vi "ScanDelay_FTIR_GetSpectrum_Aligning.vi"(0 "Cancel? External":refnum<vi>, 1 "% averaged (external)":refnum<vi>, 2 "Binned interferogram (external)":refnum<vi>, 3 "Python refnum in":refnum<k35>, 5 "Optimize\ninterferogram\ndelay":bool, 7 "Acquisition cycle (external)":refnum<vi>, 8 "Fmin / Fmax":T1={"Min frequency"=800.0, "Max frequency"=2500.0}, 9 "Displacement\n calibration  factor":dbl=-2.438, 10 "Python error in":errorcluster, 11 "Channels to read  (ScanDelay X, chan(1,2,..))":tag="Dev1/ai3,Dev1/ai2,Dev1/ai2", 12 "Acquisitions per interferogram":i32=30, 13 "Time per\nacquisition (s)":dbl=0.18, 14 "Sampling rate":dbl=250000.0, 15 "Delay estimation (pts)":i32=-10) -> (4 "Output spectrum":dbl[][](array[numeric]), 6 "Best delay":i32)   [LabVIEW 2022 SP3]
uses:
  Control_GetSpectrum_Aligning.ctl
  <vilib>/DAQmx/read.llb/DAQmx Read (Analog 2D DBL NChan NSamp).vi
  <vilib>/DAQmx/miscellaneous.llb/DAQmx Fill In Error Info.vi
panel:
  out "size(s)":i32[](array[numeric])
  out "Number of signal channels":i32
  in  "Gain":dbl=1.0
  in  "First clear existing DAQmx tasks":bool=TRUE
  in  "Optimize over delay range":i32=5
  in  "Flattening order":i32=5
  out "DAQmx error":errorcluster={"status"=FALSE, "code"=200012, "source"="DAQmx Control Task.vi:3900003"}
  out "Time per\nloop (ms)":dbl=199.0
  in  "Save interferograms\n(interferograms.txt)":bool=TRUE
  out "Own python session":bool
  in  "Extract envelope":bool=TRUE
  out "Refnum errors":errorcluster
  out "Spectrum (amplitude)":cluster{dbl[], dbl[]}[](graph)
  out "Spectrum (phase)":cluster{dbl[], dbl[]}[](graph)
  out "Interferogram (aligned)":cluster{dbl[], dbl[]}[](graph)
  out "% averaged":dbl=46.666666666666664
  out "Acquisition cycle":dbl[][](graph)
  out "Python error out":errorcluster
  in  "Halt acquisition":bool
  in  "Subtract\ndisplacement (ps)":dbl
  out "Python module path":path=path "C:/Users/mnopl/Desktop/Software/mnOPSuite/PRISM/python/scandelay_FTIR.py"
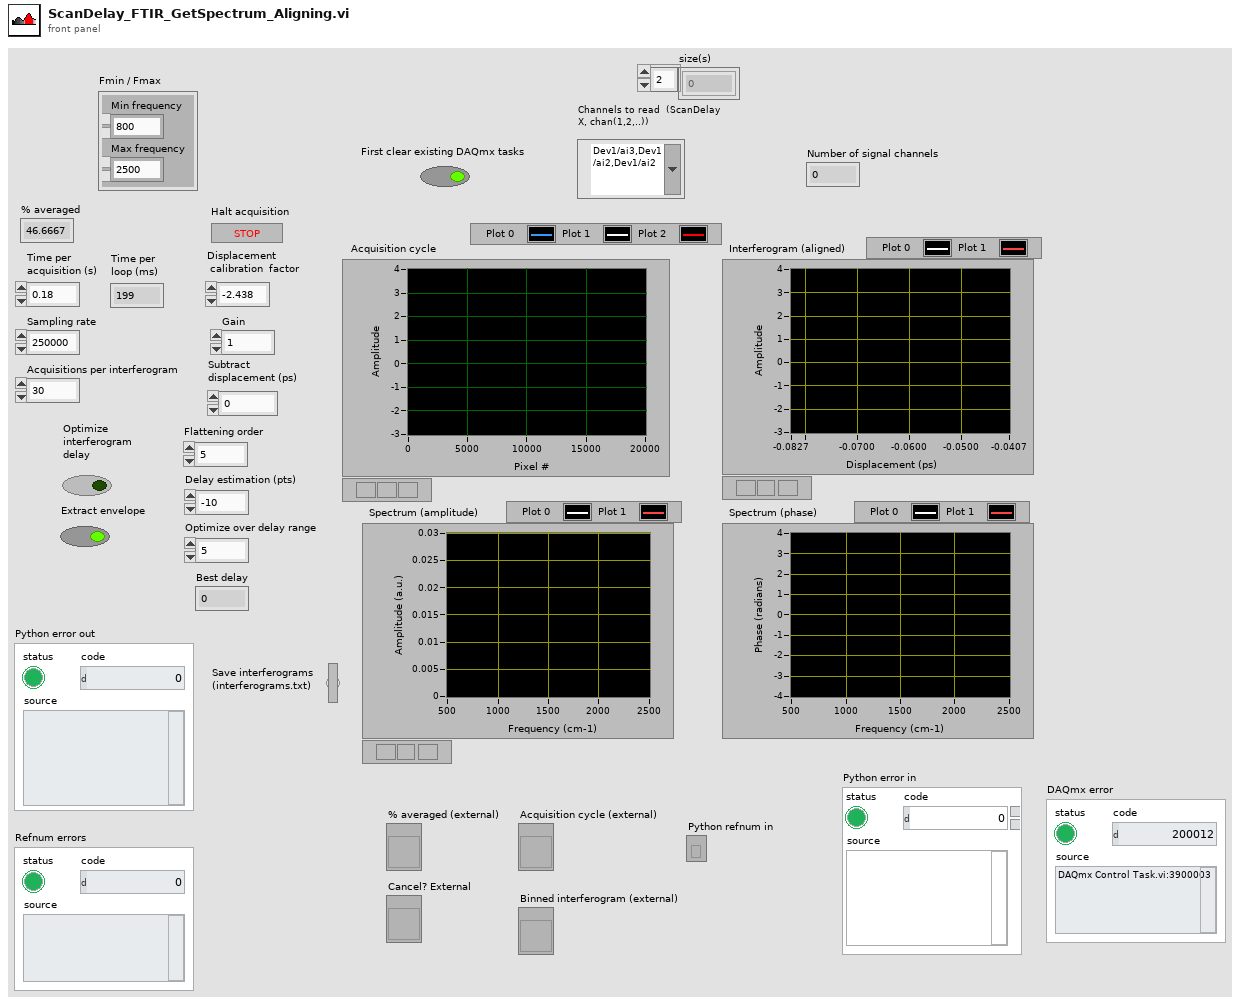
[diagram p1: front panel]
types:
  T1 = cluster{"Min frequency":dbl, "Max frequency":dbl}
  T2 = typedef "Control_GetSpectrum_Aligning.ctl" = enum16{"Acquire Interferograms", "Prepare DAQ task", "Align Interferograms", "Compute Spectrum", "Done"}
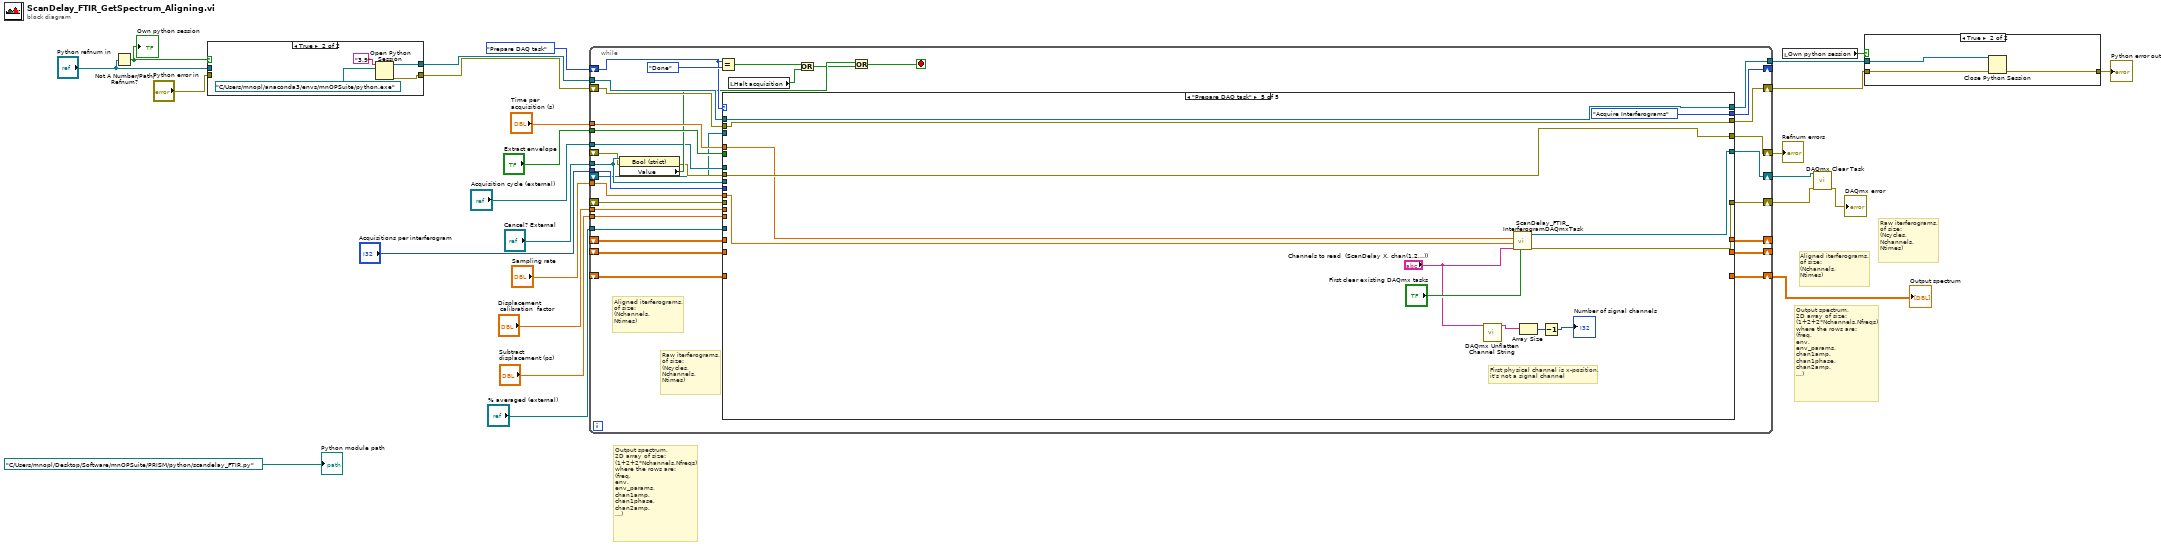
[diagram p0: block diagram]
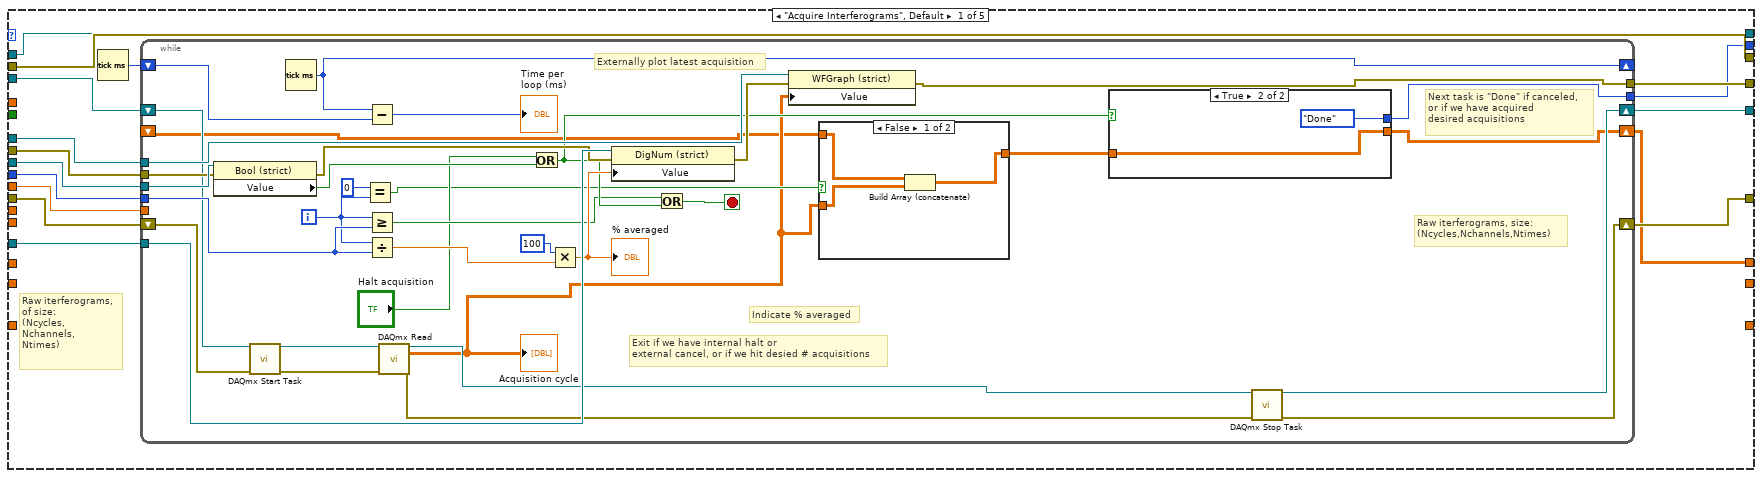
[diagram p4: hidden frame]
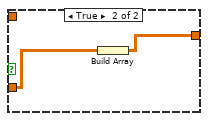
[diagram p5: hidden frame]
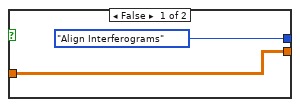
[diagram p6: hidden frame]
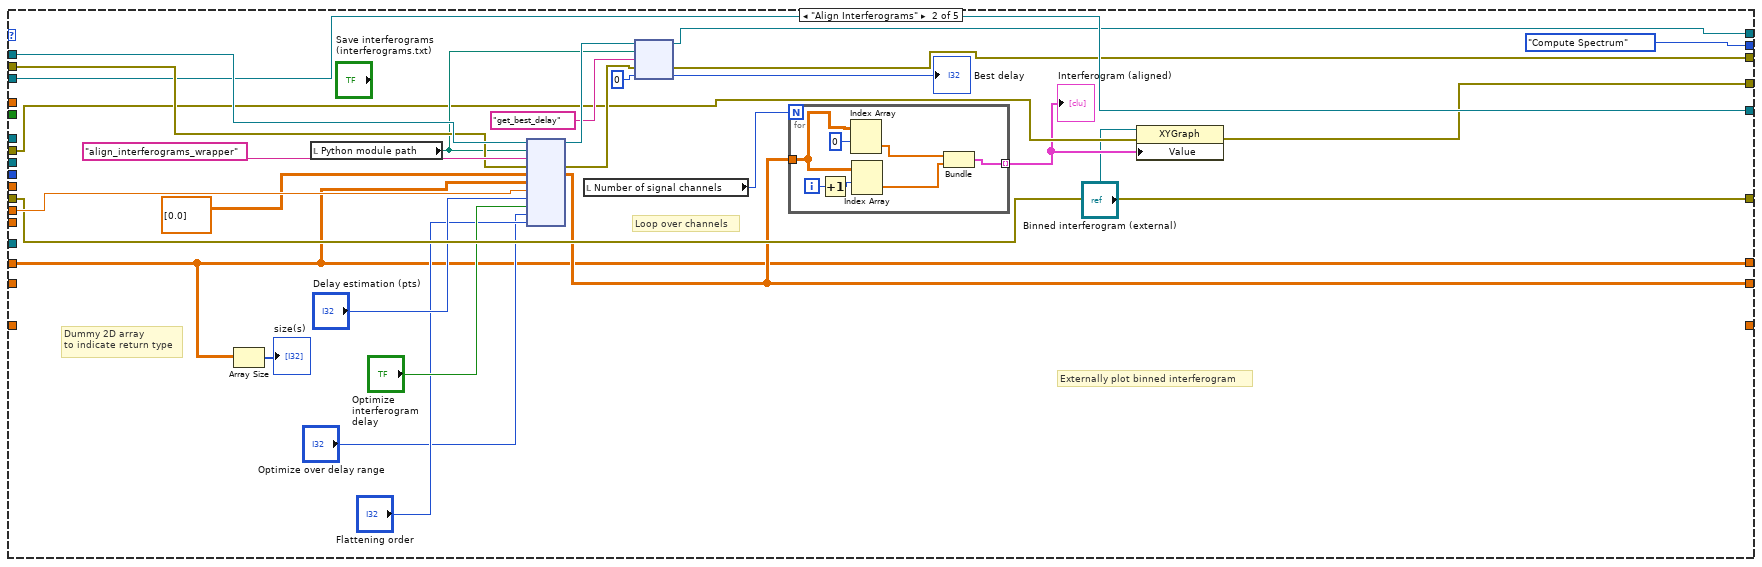
[diagram p7: hidden frame]
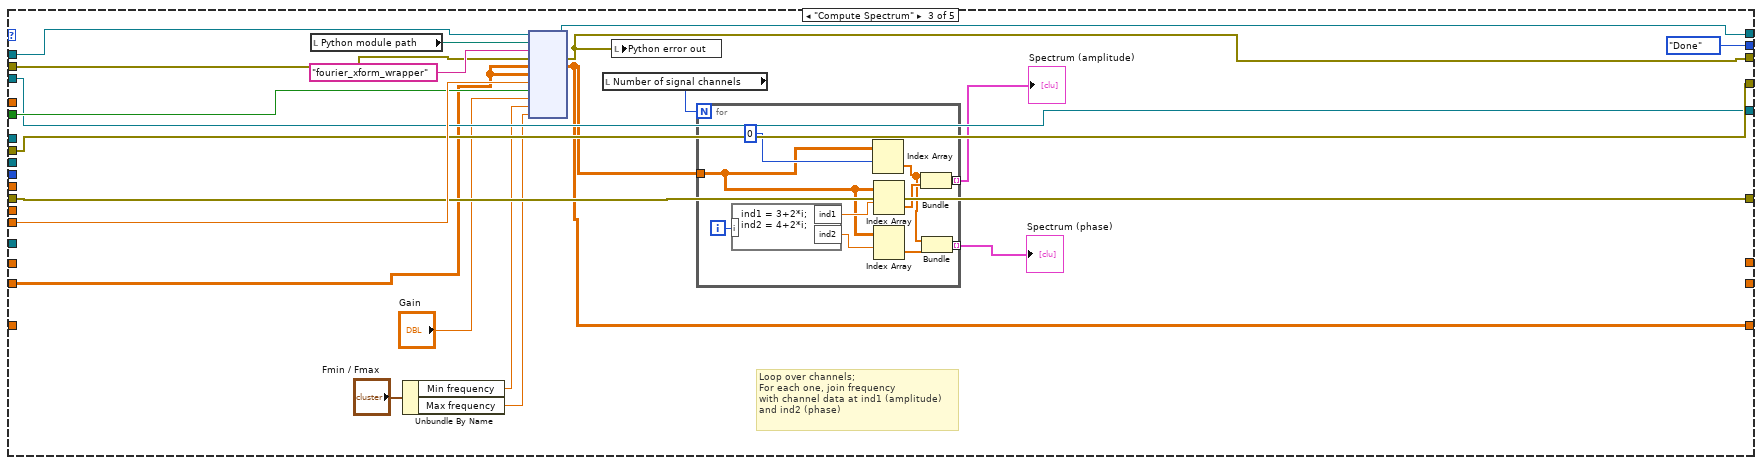
[diagram p8: hidden frame]
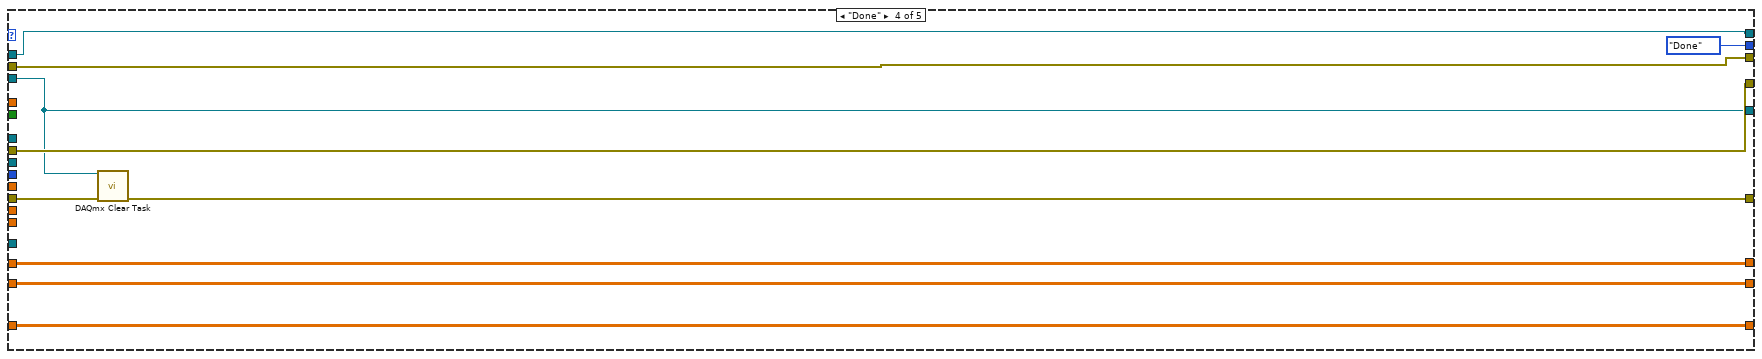
[diagram p9: hidden frame]
diagram:
  # "Output spectrum,\n2D array of size:\n(1+2+2*Nchannels,Nfreqs)\nwhere the rows are:\n(freq,\nenv,\nenv_params,\nchan1amp,\nchan1phase,\nchan2amp,\n...)"
  # "Output spectrum,\n2D array of size:\n(1+2+2*Nchannels,Nfreqs)\nwhere the rows are:\n(freq,\nenv,\nenv_params,\nchan1amp,\nchan1phase,\nchan2amp,\n...)"
  # "Aligned iterferograms,\nof size:\n(Nchannels,\nNtimes)"
  # "Raw iterferograms,\nof size:\n(Ncycles,\nNchannels,\nNtimes)"
  n1 = Not A Number/Path/Refnum?(number/path/refnum="Python refnum in") -> (NaN/Path/Refnum?=w7:bool)
  "Own python session" <- w7
  n2 = case shown="True" w7 {
    tunnel: [w27 w29] -> w11
    tunnel: [w26 w28] -> w10
    tunnel: "Python refnum in" -> [w27 _]
    tunnel: "Python error in" -> [w26 _]
    frame False {
    }
    frame True {
      n3 = Open Python Session(python version="3.9", python path=path "C:/Users/mnopl/anaconda3/envs/mnOPSuite/python.exe") -> (session out=w29:refnum<k35>, error out=w28:errorcluster)  [unwired: 1 in]
    }
  }
  n4 = while {
    tunnel: w11 -> [w65]
    tunnel: "Acquisition cycle (external)" -> [w42]
    tunnel: "Sampling rate" -> [w63]
    tunnel: "Time per\nacquisition (s)" -> [w62]
    tunnel: "Displacement\n calibration  factor" -> [w61]
    tunnel: "% averaged (external)" -> [w60]
    tunnel: "Cancel? External" -> [w45]
    tunnel: "Acquisitions per interferogram" -> [w59]
    shift-right: [w58] -> _
    shift-left: Control_GetSpectrum_Aligning."Prepare DAQ task" -> [w50]
    tunnel: "Subtract\ndisplacement (ps)" -> [w57]
    tunnel: [w54] -> w15
    shift-right: [w53] -> w14
    shift-left: w10 -> [w64]
    tunnel: "Extract envelope" -> [w52]
    shift-right: [w51] -> w12
    shift-left: _ -> [w43]
    shift-right: [w40] -> w4
    shift-left: _ -> [w38]
    shift-right: [w41] -> w2
    shift-left: _ -> [w39]
    shift-right: [w37] -> _
    shift-left: _ -> [w36]
    shift-right: [w35] -> _
    shift-left: _ -> [w34]
    shift-right: [w33] -> w1
    shift-left: _ -> [w32]
    stop <- w47 stop-if-true
    # "Aligned iterferograms,\nof size:\n(Nchannels,\nNtimes)"
    # "Raw iterferograms,\nof size:\n(Ncycles,\nNchannels,\nNtimes)"
    n5 = property on="Property Node" class="Bool (strict)"(reference=w45, error in=w43) -> (error out=w44:errorcluster, "Value"=w49:bool)  [unwired: 1 out]
    n6 = Equal?(x=w50, y=Control_GetSpectrum_Aligning."Done") -> (x = y?=w55:bool)
    n7 = case shown="\"Prepare DAQ task\"" w50 {
      tunnel: w65 -> [w68 w152 w180 w200 w210]
      tunnel: w64 -> [w77 w151 w177 w201 w209]
      tunnel: w42 -> [w81 _ _ _ _]
      tunnel: w63 -> [w80 _ _ _ w207]
      tunnel: w62 -> [_ _ _ _ w208]
      tunnel: w61 -> [_ w149 _ _ _]
      tunnel: w60 -> [w79 _ _ _ _]
      tunnel: w45 -> [w78 _ _ _ _]
      tunnel: w59 -> [w75 _ _ _ _]
      tunnel: [w68 w141 w179 w200 w210] -> w54
      tunnel: [w73 Control_GetSpectrum_Aligning."Compute Spectrum" Control_GetSpectrum_Aligning."Done" Control_GetSpectrum_Aligning."Done" Control_GetSpectrum_Aligning."Acquire Interferograms"] -> w58
      tunnel: w57 -> [_ _ w176 _ _]
      tunnel: [w77 w139 w173 w201 w209] -> w53
      tunnel: w52 -> [_ _ w174 _ _]
      tunnel: [w76 w131 w172 w198 w212] -> w51
      tunnel: w44 -> [w74 w132 w172 w198 w212]
      tunnel: [w70 w148 w171 w197 w214] -> w41
      tunnel: [w69 w147 w170 w195 w213] -> w40
      tunnel: w39 -> [w72 w148 w171 w197 _]
      tunnel: w38 -> [w71 w147 w170 w196 _]
      tunnel: [w66 w127 _ w192 _] -> w37
      tunnel: w36 -> [_ w127 _ w192 _]
      tunnel: [_ w133 _ w193 _] -> w35
      tunnel: w34 -> [_ _ w165 w193 _]
      tunnel: [_ _ w164 w194 _] -> w33
      tunnel: w32 -> [_ _ _ w194 _]
      frame "Acquire Interferograms", Default {
        # "Raw iterferograms,\nof size:\n(Ncycles,\nNchannels,\nNtimes)"
        n8 = Tick Count (ms)() -> (millisecond timer value=w67:u32)
        n9 = while {
          tunnel: w81 -> [w112]
          tunnel: w80 -> [_]
          tunnel: w79 -> [w114]
          tunnel: w78 -> [w109]
          tunnel: [w110] -> w76
          shift-right: [w88] -> w66
          shift-left: _ -> [w83]
          tunnel: w75 -> [w103]
          tunnel: w74 -> [w108]
          tunnel: [w105] -> w73
          shift-right: [w100] -> w70
          shift-left: w72 -> [w91]
          shift-right: [w101] -> w69
          shift-left: w71 -> [w90]
          shift-right: [w99] -> _
          shift-left: w67 -> [w98]
          i -> [w87]
          stop <- w106 stop-if-true
          # "Raw iterferograms, size:\n(Ncycles,Nchannels,Ntimes)"
          # "Next task is \"Done\" if canceled,\nor if we have acquired \ndesired acquisitions"
          # "Exit if we have internal halt or\nexternal cancel, or if we hit desied # acquisitions"
          # "Externally plot latest acquisition"
          # "Indicate % averaged"
          n10 = property on="Property Node" class="Bool (strict)"(reference=w109, error in=w108) -> (error out=w107:errorcluster, "Value"=w104:bool)  [unwired: 1 out]
          n11 = call <vilib>:"DAQmx Start Task.vi"("task/channels in"=w91, "error in"=w90) -> ("task out"=w92:refnum<k21>, "error out"=w89:errorcluster)  [unwired: 12 in]
          n12 = Tick Count (ms)() -> (millisecond timer value=w99:u32)
          n13 = Equal?(x=0, y=w87) -> (x = y?=w85:bool)
          n14 = Subtract(x=w99, y=w98) -> (x-y=→"Time per\nloop (ms)":u32)
          n15 = Greater Or Equal?(x=w87, y=w103) -> (x >= y?=w95:bool)
          n16 = Divide(x=w87, y=w103) -> (x/y=w116:dbl)
          n17 = call-poly <vilib>:"DAQmx Read.vi"("task/channels in"=w92, "error in"=w89) -> ("task out"=w93:refnum<k21>, "data"=w84:dbl[][], "error out"=w102:errorcluster)  [unwired: 11 in]
          "Acquisition cycle" <- w84
          n18 = Or(x="Halt acquisition", y=w104) -> (x .or. y?=w96:bool)
          n19 = Multiply(x=100, y=w116) -> (x*y=w113:dbl)
          "% averaged" <- w113
          n20 = property on="Property Node" class="DigNum (strict)"(reference=w114, error in=w107, "Value"=w113) -> (error out=w111:errorcluster)  [unwired: 1 out]
          n21 = Or(x=w95, y=w96) -> (x .or. y?=w106:bool)
          n22 = property on="Property Node" class="WFGraph (strict)"(reference=w112, error in=w111, "Value"=w84) -> (error out=w110:errorcluster)  [unwired: 1 out]
          n23 = case shown="False" w85 {
            tunnel: w84 -> [w118 w121]
            tunnel: w83 -> [w119 _]
            tunnel: [w117 w120] -> w82
            frame False {
              n24 = Build Array (concatenate)(w119, w118) -> (w117:dbl[][][])
            }
            frame True {
              n25 = Build Array(w121) -> (w120:dbl[][][])
            }
          }
          n26 = case shown="True" w96 {
            tunnel: [Control_GetSpectrum_Aligning."Align Interferograms" Control_GetSpectrum_Aligning."Done"] -> w105
            tunnel: [w122 w124] -> w88
            tunnel: w82 -> [w122 w124]
            frame False {
            }
            frame True {
            }
          }
          n27 = call <vilib>:"DAQmx Stop Task.vi"("task/channels in"=w93, "error in"=w102) -> ("task out"=w100:refnum<k21>, "error out"=w101:errorcluster)  [unwired: 12 in]
        }
      }
      frame "Align Interferograms" {
        # "Loop over channels"
        # "Dummy 2D array\nto indicate return type"
        # "Externally plot binned interferogram"
        n28 = Array Size(array=w127) -> (size(s)=→"size(s)":i32[])
        n29 = local read "Python module path"() -> (w138:path)
        n30 = node(w152, w138, "align_interferograms_wrapper", w151, dbl[][] [[0.0]], w127, w149, "Delay estimation (pts)", "Optimize\ninterferogram\ndelay", "Optimize over delay range", "Flattening order") -> (w142:refnum<k35>, w140:errorcluster, w133:dbl[][])  [unwired: 6 in, 2 out]
        n31 = local read "Number of signal channels"() -> (w128:i32)
        n32 = node(w142, w138, "get_best_delay", w140, 0) -> (w141:refnum<k35>, w139:errorcluster, →"Best delay":i32)  [unwired: 2 out]
        n33 = for {
          N: w128 -> [_]
          tunnel: [w156] -> w130 mode=indexing
          tunnel: w133 -> [w159]
          i -> [w155]
          n34 = Increment(x=w155) -> (x+1=w154:i32)
          n35 = Index Array(array=w159, index (row)=0 ("index")) -> (element=w158:dbl[])  [unwired: 1 in]
          n36 = Index Array(array=w159, index (row)=w154) -> (element=w157:dbl[])  [unwired: 1 in]
          n37 = Bundle(w158, w157) -> (w156:cluster{dbl[], dbl[]})  [unwired: 1 in]
        }
        "Interferogram (aligned)" <- w130
        n38 = property class="XYGraph"(reference="Binned interferogram (external)", error in=w132, "Value"=w130) -> (error out=w131:errorcluster)  [unwired: 1 out]
      }
      frame "Compute Spectrum" {
        # "Loop over channels;\nFor each one, join frequency\nwith channel data at ind1 (amplitude)\nand ind2 (phase)"
        n39 = local read "Python module path"() -> (w178:path)
        n40 = Unbundle By Name("Fmin / Fmax") -> ("Min frequency"=w166:dbl, "Max frequency"=w167:dbl)
        n41 = node(w180, w178, "fourier_xform_wrapper", w177, w165, w165, w176, w174, "Gain", w166, w167) -> (w179:refnum<k35>, w173:errorcluster, w164:dbl[][])  [unwired: 6 in, 2 out]
        n42 = local read "Number of signal channels"() -> (w163:i32)
        n43 = local write "Python error out"(w173) -> ()
        n44 = for {
          N: w163 -> [_]
          tunnel: w164 -> [w186]
          tunnel: [w183] -> w162 mode=indexing
          tunnel: [w182] -> w161 mode=indexing
          i -> [w189]
          n45 = formula code="ind1 = 3+2*i;\nind2 = 4+2*i;"("i"=w189) -> ("ind1"=w188:dbl, "ind2"=w187:dbl)
          n46 = Index Array(array=w186, index (row)=0) -> (element=w185:dbl[])  [unwired: 1 in]
          n47 = Index Array(array=w186, index (row)=w188) -> (element=w191:dbl[])  [unwired: 1 in]
          n48 = Index Array(array=w186, index (row)=w187) -> (element=w184:dbl[])  [unwired: 1 in]
          n49 = Bundle(w185, w191) -> (w183:cluster{dbl[], dbl[]})  [unwired: 1 in]
          n50 = Bundle(w185, w184) -> (w182:cluster{dbl[], dbl[]})  [unwired: 1 in]
        }
        "Spectrum (phase)" <- w161
        "Spectrum (amplitude)" <- w162
      }
      frame "Done" {
        n51 = call <vilib>:"DAQmx Clear Task.vi"("task in"=w197, "error in"=w196) -> ("error out"=w195:errorcluster)  [unwired: 13 in]
      }
      frame "Prepare DAQ task" {
        # "First physical channel is x-position,\nit's not a signal channel"
        n52 = call <vilib>:"DAQmx Unflatten Channel String.vi"("names in"="Channels to read  (ScanDelay X, chan(1,2,..))") -> ("names out"=w204:string[])  [unwired: 13 in, 1 out]
        n53 = call "ScanDelay_FTIR_InterferogramDAQmxTask.vi"("First clear existing DAQmx tasks"="First clear existing DAQmx tasks", "Channels to read"="Channels to read  (ScanDelay X, chan(1,2,..))", "Sampling rate"=w207, "Time per acquisiton (s)"=w208) -> ("error out"=w213:errorcluster, "Refnum out"=w214:refnum<k21>)  [unwired: 6 in]
        n54 = Array Size(array=w204) -> (size(s)=w203:i32)
        n55 = Decrement(x=w203) -> (x-1=→"Number of signal channels":i32)
      }
    }
    n56 = local read "Halt acquisition"() -> (w46:bool)
    n57 = Or(x=w55, y=w46) -> (x .or. y?=w48:bool)
    n58 = Or(x=w49, y=w48) -> (x .or. y?=w47:bool)
  }
  "Output spectrum" <- w1
  "Refnum errors" <- w12
  n59 = local read "Own python session"() -> (w6:bool)
  n60 = call <vilib>:"DAQmx Clear Task.vi"("task in"=w2, "error in"=w4) -> ("error out"=→"DAQmx error":errorcluster)  [unwired: 13 in]
  n61 = case shown="True" w6 {
    tunnel: [w215 w218] -> w16
    tunnel: w15 -> [_ w217]
    tunnel: w14 -> [w215 w216]
    frame False {
    }
    frame True {
      n62 = Close Python Session(session in=w217, error in=w216) -> (11:w218:errorcluster)
    }
  }
  "Python error out" <- w16
  "Python module path" <- path "C:/Users/mnopl/Desktop/Software/mnOPSuite/PRISM/python/scandelay_FTIR.py"
